vi "Teleop.vi"(10 "Match Info":T1={"Autonomous Elapsed Seconds"=0.0, "TeleOp Elapsed Seconds"=0.0, "Disabled Elapsed Seconds"=0.0, "Visited Autonomous"=FALSE, "Visited TeleOp"=FALSE, "Visited Disabled"=FALSE, "Autonomous Settings"={"Autonomous Style"=enum."Independent", "VI Refnum"=refnum}}, 11 "Call Context":T2) -> ()   [LabVIEW 2016]
doc: "This VI is called for each TeleOp packet received from the DS where the robot is not disabled. It is often used to read from the joysticks and update I/O or to update setpoints for timed control loops. It should complete and return within 20 milliseconds or it may miss DS packets."
uses:
  <vilib>/Rock Robotics/WPI/DriverStation/WPI_DriverStationDerivedRobotMode.ctl
  <vilib>/Rock Robotics/WPI/DriverStation/WPI_DriverStationMatch Info.ctl
  <vilib>/Rock Robotics/WPI/Utilities/WPI_GetSetVariantRefNum.vi
  Encoder Rate Shooter.vi
  <vilib>/Rock Robotics/Network Tables/NT Write Boolean Array.vi
  <vilib>/Rock Robotics/Network Tables/NT Write Numeric Array.vi
  <vilib>/Rock Robotics/WPI/RobotDrive/WPI_RobotDriveMecanumDrive_Cartesian.vi
panel:
  out "Init Encoder":bool
  out "Rotation":dbl
  out "Y":dbl
  out "X":dbl
  in  "Shooter Control":dbl
  out "Boolean":bool
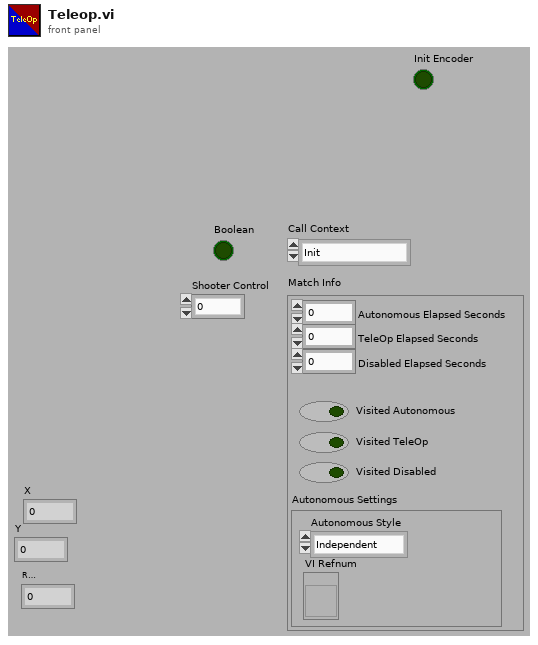
[diagram p1: front panel]
types:
  T1 = typedef "WPI_DriverStationMatch Info.ctl" = cluster{"Autonomous Elapsed Seconds":dbl, "TeleOp Elapsed Seconds":dbl, "Disabled Elapsed Seconds":dbl, "Visited Autonomous":bool, "Visited TeleOp":bool, "Visited Disabled":bool, "Autonomous Settings":cluster{"Autonomous Style":enum16{"Iterative", "Independent"}, "VI Refnum":refnum<vi>}}
  T2 = typedef "WPI_DriverStationDerivedRobotMode.ctl" = enum16{"Init", "Execute", "Stop"}
  T3 = typedef "WPI_JoystickDevRef.ctl" = cluster{"Device":T4}
  T4 = typedef "WPI_JoystickDeviceEnum.ctl" = enum16{"USB 0", "USB 1", "USB 2", "USB 3", "USB 4", "USB 5"}
  T5 = typedef "WPI_MotorControlDeviceRef.ctl" = cluster{"DeviceStatus":errorcluster, "Type":T6, "PWM":cluster{"PWM Channel":T7, "DeadBand":T8}, "CAN":cluster{"Device Number":u8, "SetOutput VI Ref":variant, "GetOutput VI Ref":variant, "Enable VI Ref":variant, "Disable VI Ref":variant, "Data":variant}, "Invert":bool}
  T6 = typedef "WPI_MotorControlType.ctl" = enum16{"PWM", "CAN"}
  T7 = typedef "FPGA_DIOPWMChannel.ctl" = enum8{"PWM 0", "PWM 1", "PWM 2", "PWM 3", "PWM 4", "PWM 5", "PWM 6", "PWM 7", "PWM 8", "PWM 9", "PWM MXP 0", "PWM MXP 1", "PWM MXP 2", "PWM MXP 3", "PWM MXP 4", "PWM MXP 5", "PWM MXP 6", "PWM MXP 7", "PWM MXP 8", "PWM MXP 9", "Invalid"}
  T8 = typedef "WPI_PWMDeadband.ctl" = cluster{"Name":string, "maxPositivePwm":i32, "minPositivePwm":i32, "centerPwm":i32, "maxNegativePwm":i32, "minNegativePwm":i32, "angularRange":u16}
  T9 = typedef "WPI_RobotDriveDevRef.ctl" = cluster{"DevStatus":errorcluster, "Motors[]":T5[], "Square Inputs":bool, "Max Output":dbl}
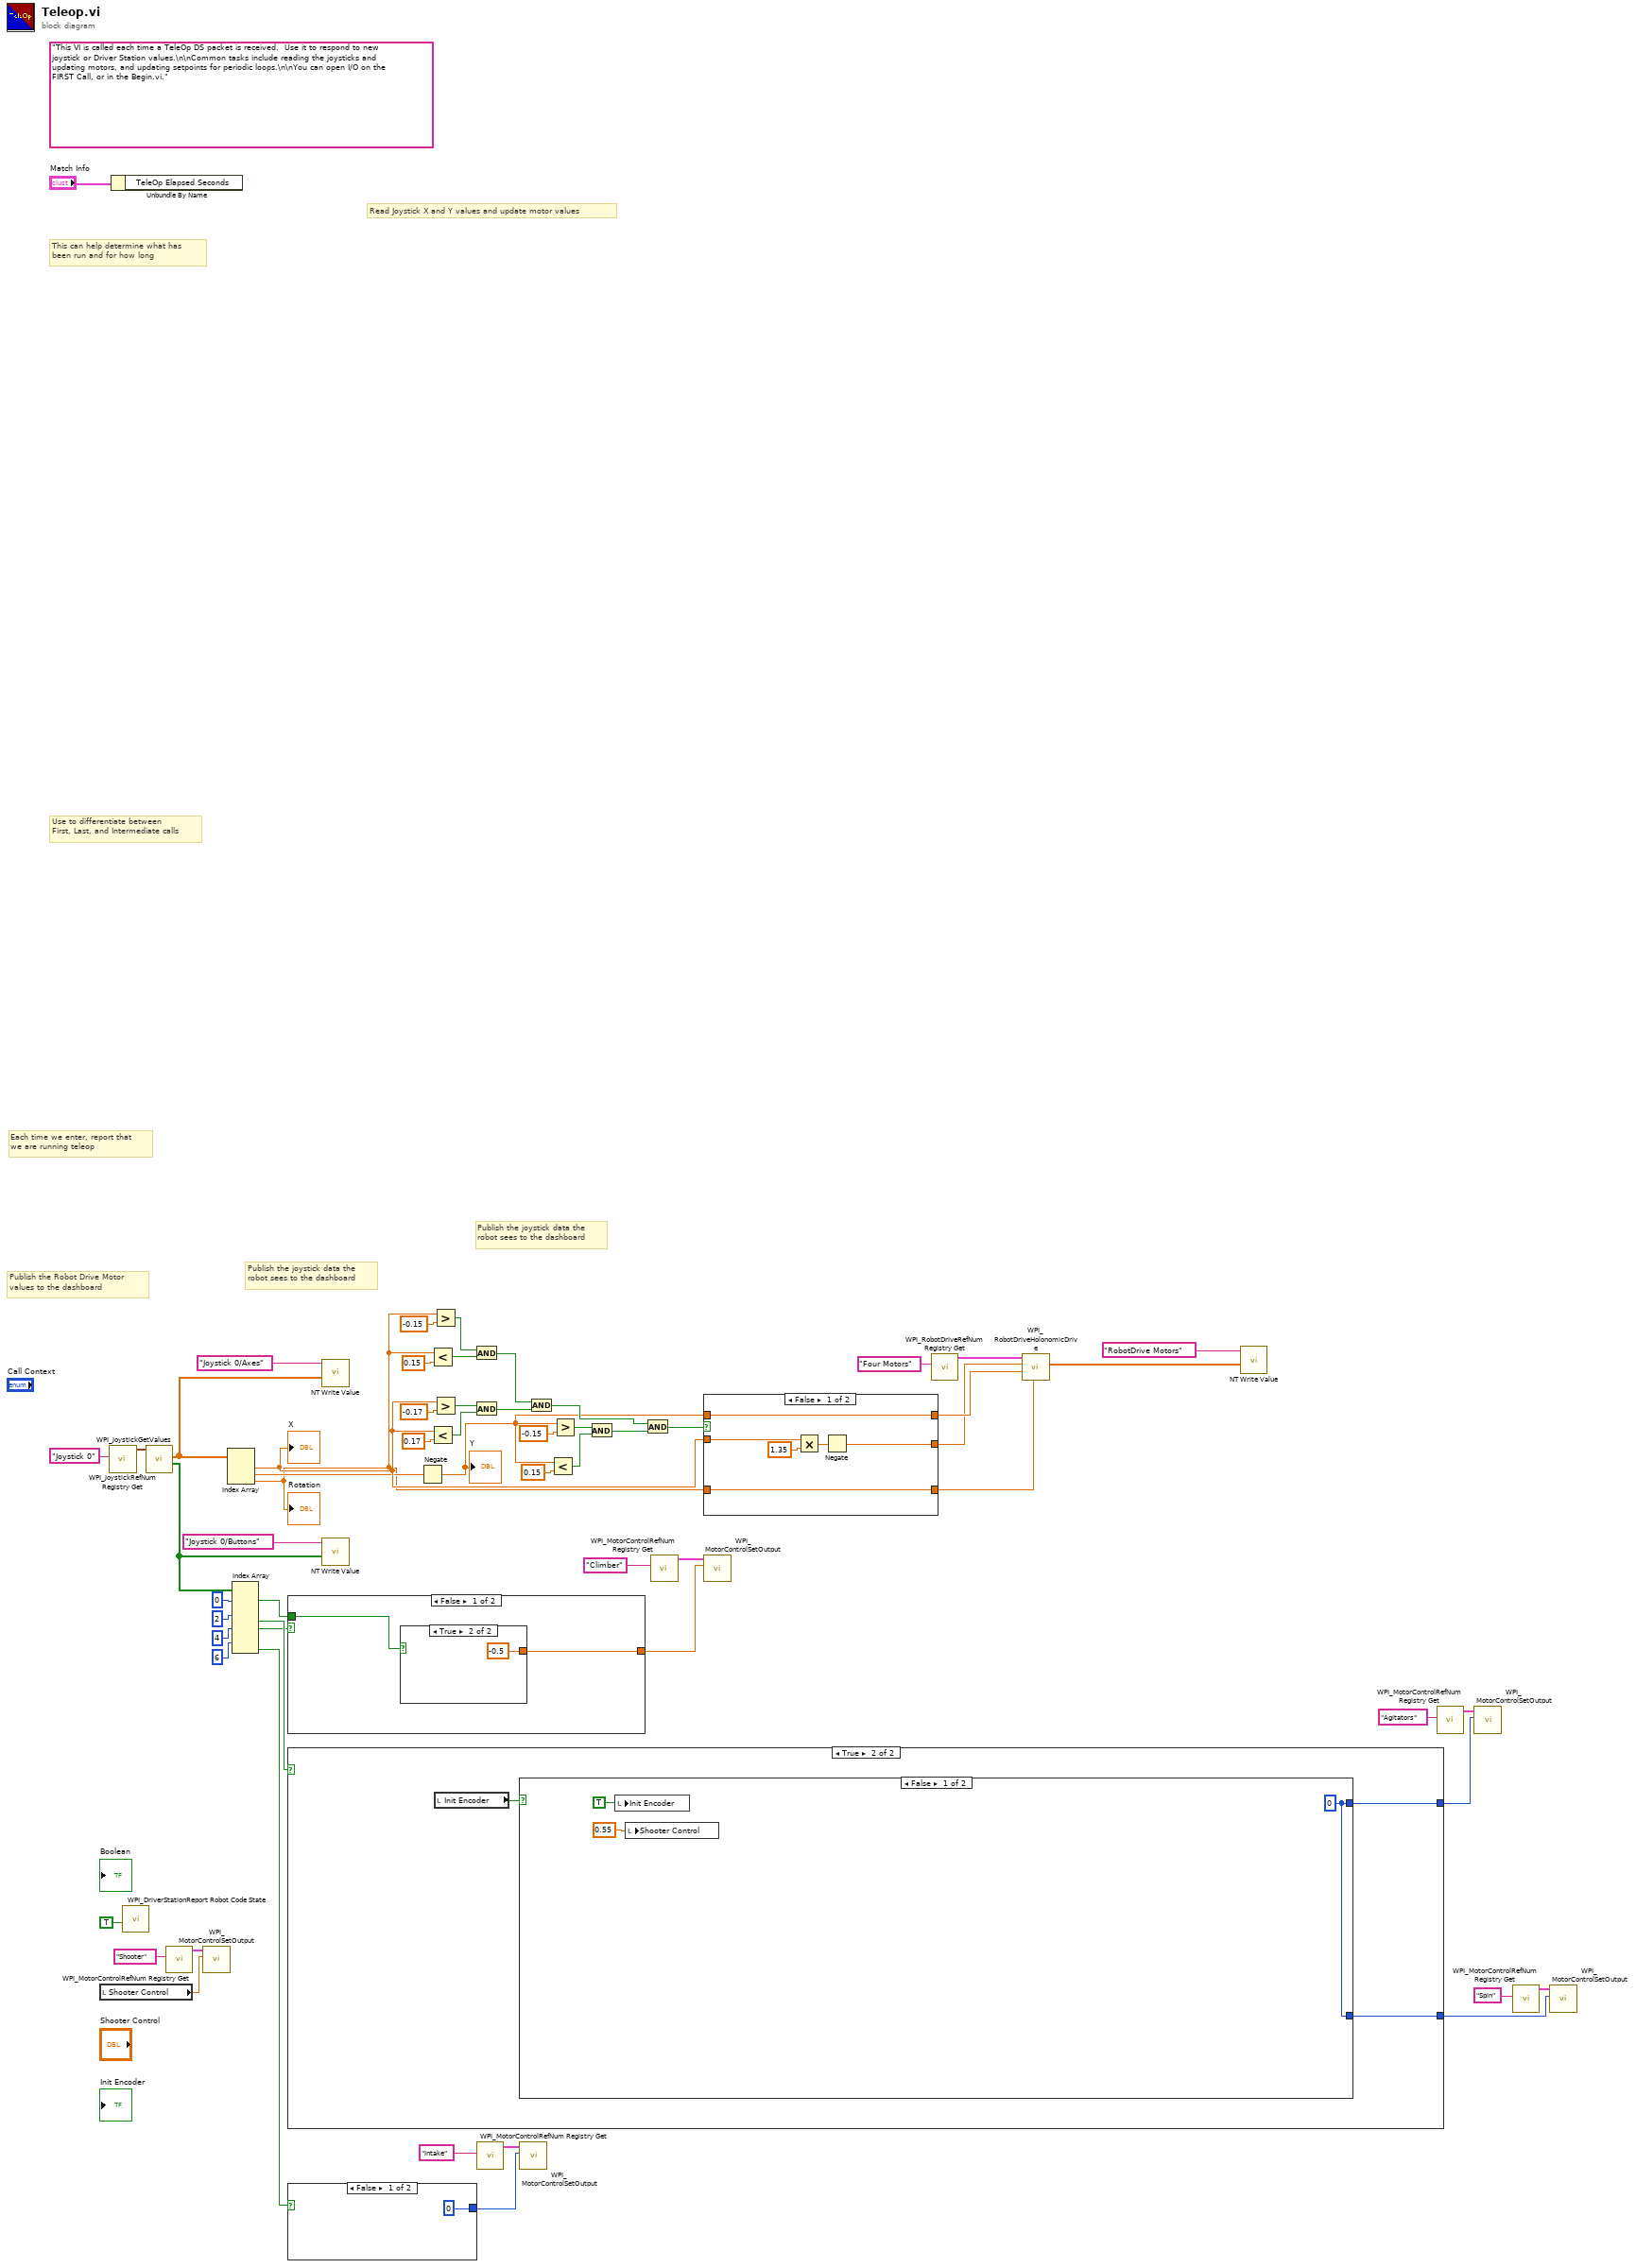
[diagram p0: block diagram]
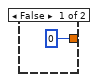
[diagram p2: hidden frame]
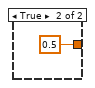
[diagram p3: hidden frame]
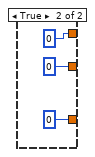
[diagram p4: hidden frame]
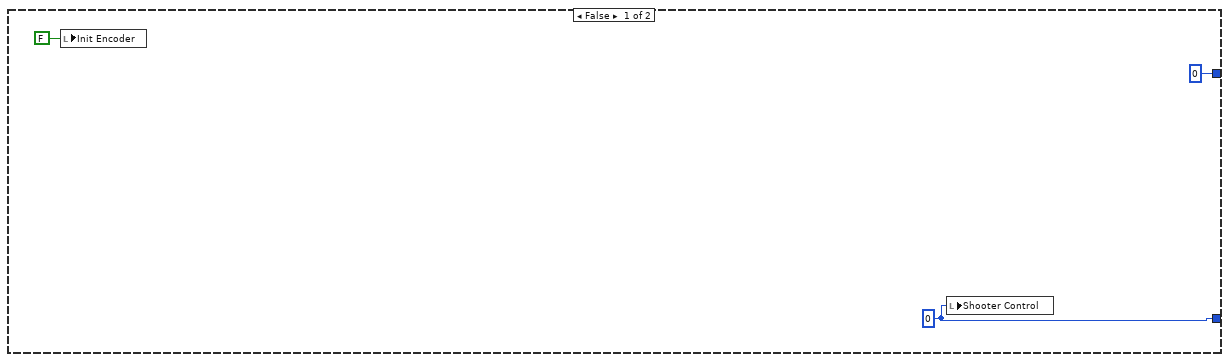
[diagram p5: hidden frame]
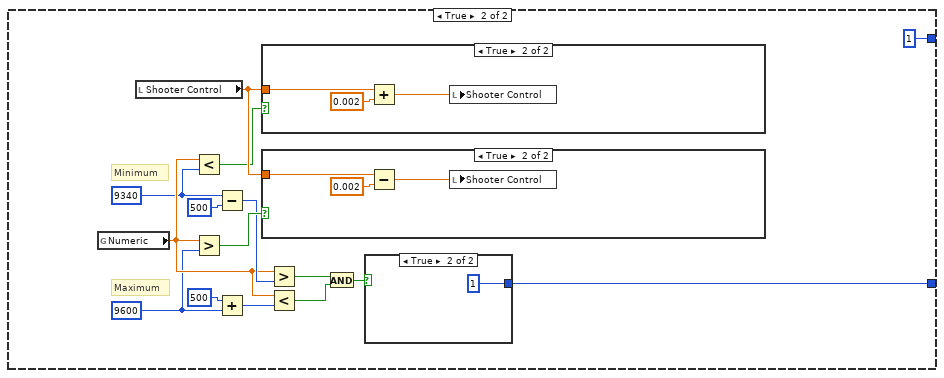
[diagram p6: hidden frame]
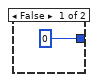
[diagram p7: hidden frame]
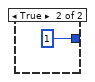
[diagram p10: hidden frame]
diagram:
  (unwired) "This VI is called each time a TeleOp DS packet is received.  Use it to respond to new joystick or Driver Station values.\n\nCommon tasks include reading the joysticks and updating motors, and updating setpoints for periodic loops.\n\nYou can open I/O on the FIRST Call, or in the Begin.vi."
  # "Publish the joystick data the\nrobot sees to the dashboard"
  # "Publish the Robot Drive Motor\nvalues to the dashboard"
  # "Publish the joystick data the\nrobot sees to the dashboard"
  # "Each time we enter, report that\nwe are running teleop"
  # "Use to differentiate between\nFirst, Last, and Intermediate calls"
  # "This can help determine what has\nbeen run and for how long"
  # "Read Joystick X and Y values and update motor values"
  n1 = local read "Shooter Control"() -> (w50:dbl)
  n2 = call <vilib>:"WPI_JoystickRefNum Registry Get.vi"("refnum name"="Joystick 0") -> ("JoystickDevRef"=w44:T3)  [unwired: 1 in, 9 out]
  n3 = Unbundle By Name("Match Info") -> ()  [unwired: 1 out]
  n4 = call <vilib>:"WPI_DriverStationReport Robot Code State.vi"("TeleOp"=TRUE ("Autonomous")) -> ()  [unwired: 10 in, 1 out]
  n5 = call <vilib>:"WPI_JoystickGetValues.vi"("JoystickDevRef"=w44) -> ("Buttons"=w38:bool[], "Axes"=w42:dbl[])  [unwired: 6 in, 3 out]
  n6 = call <vilib>:"WPI_MotorControlRefNum Registry Get.vi"("refnum name"="Shooter") -> ("MotorControlDevRef"=w52:T5)  [unwired: 9 in, 1 out]
  n7 = call <vilib>:"WPI_MotorControlSetOutput.vi"("Output"=w50, "MotorControlDevRef"=w52) -> ()  [unwired: 7 in, 3 out]
  n8 = Index Array(array=w42) -> (element #1=w29:dbl, element #2=w4:dbl, element #3=w1:dbl)  [unwired: 3 in]
  "X" <- w29
  "Rotation" <- w1
  n9 = Index Array(array=w38, index #1=0, index #3=2, index #5=4, index #7=6) -> (element #1=w12:bool, element #4=w37:bool, element #5=w13:bool, element #8=w36:bool)  [unwired: 4 in, 4 out]
  n10 = case shown="False" w13 {
    tunnel: w12 -> [w61 _]
    tunnel: [w60 0.5] -> w11
    frame False {
      n11 = case shown="True" w61 {
        tunnel: [0 -0.5] -> w60
        frame False {
        }
        frame True {
        }
      }
    }
    frame True {
    }
  }
  n12 = case shown="True" w37 {
    tunnel: [w65 w69] -> w3
    tunnel: [0 w70] -> w2
    frame False {
      w65 = 0
      n13 = local write "Init Encoder"(FALSE) -> ()
      n14 = local write "Shooter Control"(w65) -> ()
    }
    frame True {
      n15 = local read "Init Encoder"() -> (w68:bool)
      n16 = case shown="False" w68 {
        tunnel: [w72 w86] -> w69
        tunnel: [w72 1] -> w70
        frame False {
          w72 = 0
          n17 = local write "Init Encoder"(TRUE) -> ()
          n18 = local write "Shooter Control"(0.55) -> ()
        }
        frame True {
          w74 = 9600
          w75 = 9340
          # "Minimum"
          # "Maximum"
          n19 = global read "Encoder Rate Shooter.vi" "Numeric"() -> (w77:dbl)
          n20 = local read "Shooter Control"() -> (w88:dbl)
          n21 = Less?(x=w77, y=w75) -> (x < y?=w85:bool)
          n22 = Greater?(x=w77, y=w74) -> (0:w84:bool)
          n23 = Subtract(x=w75, y=500) -> (x-y=w81:i32)
          n24 = Add(x=500, y=w74) -> (x+y=w80:i32)
          n25 = case shown="True" w85 {
            tunnel: w88 -> [_ w95]
            frame False {
            }
            frame True {
              n26 = Add(x=w95, y=0.002) -> (x+y=w94:dbl)
              n27 = local write "Shooter Control"(w94) -> ()
            }
          }
          n28 = case shown="True" w84 {
            tunnel: w88 -> [_ w92]
            frame False {
            }
            frame True {
              n29 = Subtract(x=w92, y=0.002) -> (x-y=w91:dbl)
              n30 = local write "Shooter Control"(w91) -> ()
            }
          }
          n31 = Greater?(x=w77, y=w81) -> (0:w78:bool)
          n32 = Less?(x=w77, y=w80) -> (x < y?=w79:bool)
          n33 = And(x=w78, y=w79) -> (x .and. y?=w87:bool)
          n34 = case shown="True" w87 {
            tunnel: [0 1] -> w86
            frame False {
            }
            frame True {
            }
          }
        }
      }
    }
  }
  n35 = case shown="False" w36 {
    tunnel: [0 1] -> w54
    frame False {
    }
    frame True {
    }
  }
  n36 = call-poly <vilib>:"NT Write Value.vi"("Numeric Array"=w42, "Name"="Joystick 0/Axes") -> ()  [unwired: 9 in, 1 out]
  n37 = call-poly <vilib>:"NT Write Value.vi"("Boolean Array"=w38, "Name"="Joystick 0/Buttons") -> ()  [unwired: 9 in, 1 out]
  n38 = Negate(x=w4) -> (-x=w14:dbl)
  "Y" <- w14
  n39 = Less?(x=w1, y=0.15) -> (x < y?=w27:bool)
  n40 = Less?(x=w29, y=0.17) -> (x < y?=w32:bool)
  n41 = Greater?(x=w1, y=-0.15) -> (0:w28:bool)
  n42 = Greater?(x=w29, y=-0.17) -> (0:w33:bool)
  n43 = And(x=w28, y=w27) -> (x .and. y?=w20:bool)
  n44 = And(x=w33, y=w32) -> (x .and. y?=w19:bool)
  n45 = call <vilib>:"WPI_MotorControlRefNum Registry Get.vi"("refnum name"="Intake") -> ("MotorControlDevRef"=w57:T5)  [unwired: 9 in, 1 out]
  n46 = call <vilib>:"WPI_MotorControlSetOutput.vi"("Output"=w54, "MotorControlDevRef"=w57) -> ()  [unwired: 7 in, 3 out]
  n47 = And(x=w20, y=w19) -> (x .and. y?=w18:bool)
  n48 = Less?(x=w14, y=0.15) -> (x < y?=w23:bool)
  n49 = Greater?(x=w14, y=-0.15) -> (0:w24:bool)
  n50 = And(x=w24, y=w23) -> (x .and. y?=w17:bool)
  n51 = And(x=w18, y=w17) -> (x .and. y?=w16:bool)
  n52 = call <vilib>:"WPI_MotorControlRefNum Registry Get.vi"("refnum name"="Climber") -> ("MotorControlDevRef"=w34:T5)  [unwired: 9 in, 1 out]
  n53 = case shown="False" w16 {
    tunnel: [w102 0] -> w6
    tunnel: [w101 0] -> w5
    tunnel: [w104 0] -> w15
    tunnel: w29 -> [w103 _]
    tunnel: w1 -> [w104 _]
    tunnel: w14 -> [w102 _]
    frame False {
      n54 = Multiply(x=w103, y=1.35) -> (x*y=w100:dbl)
      n55 = Negate(x=w100) -> (-x=w101:dbl)
    }
    frame True {
    }
  }
  n56 = call <vilib>:"WPI_MotorControlSetOutput.vi"("Output"=w11, "MotorControlDevRef"=w34) -> ()  [unwired: 7 in, 3 out]
  n57 = call <vilib>:"WPI_RobotDriveRefNum Registry Get.vi"("refnum name"="Four Motors") -> ("RobotDriveDevRef"=w46:T9)  [unwired: 1 in, 9 out]
  n58 = call-poly <vilib>:"WPI_RobotDriveHolonomicDrive.vi"("Rotation"=w15, "Y"=w6, "X"=w5, "RobotDriveDevRef"=w46) -> ("Motor Values"=w39:dbl[])  [unwired: 5 in, 2 out]
  n59 = call-poly <vilib>:"NT Write Value.vi"("Numeric Array"=w39, "Name"="RobotDrive Motors") -> ()  [unwired: 9 in, 1 out]
  n60 = call <vilib>:"WPI_MotorControlRefNum Registry Get.vi"("refnum name"="Agitators") -> ("MotorControlDevRef"=w8:T5)  [unwired: 9 in, 1 out]
  n61 = call <vilib>:"WPI_MotorControlSetOutput.vi"("Output"=w2, "MotorControlDevRef"=w8) -> ()  [unwired: 7 in, 3 out]
  n62 = call <vilib>:"WPI_MotorControlRefNum Registry Get.vi"("refnum name"="Spin") -> ("MotorControlDevRef"=w10:T5)  [unwired: 9 in, 1 out]
  n63 = call <vilib>:"WPI_MotorControlSetOutput.vi"("Output"=w3, "MotorControlDevRef"=w10) -> ()  [unwired: 7 in, 3 out]
